vi "IVCurveCustom.vi"(7 "OriginalSweepInfo":T1, 8 "ReadExtra":bool=TRUE, 9 "SweepInfo":T1, 10 "Program":string, 11 "UiDefinition":T4) -> (1 "appended array":dbl[][](array[numeric]), 3 "InfoCluster":T2)   [LabVIEW 2020]
uses:
  UIReferences.ctl
  D:/LabviewDXFViewer/LabviewDXFViewer/bin/Release/LabviewDXFViewer.exe
  LabviewDXFViewer/bin/Release/LabviewDXFViewer.exe
  CapacitanceInfos.ctl
  CapacitanceRecord.ctl
  Keithley 2600 Series/Keithley 2600 Series.lvlib
panel:
  out "error out 4":errorcluster
  out "error out 3":errorcluster
  out "error out 2":errorcluster
  out "error out":errorcluster
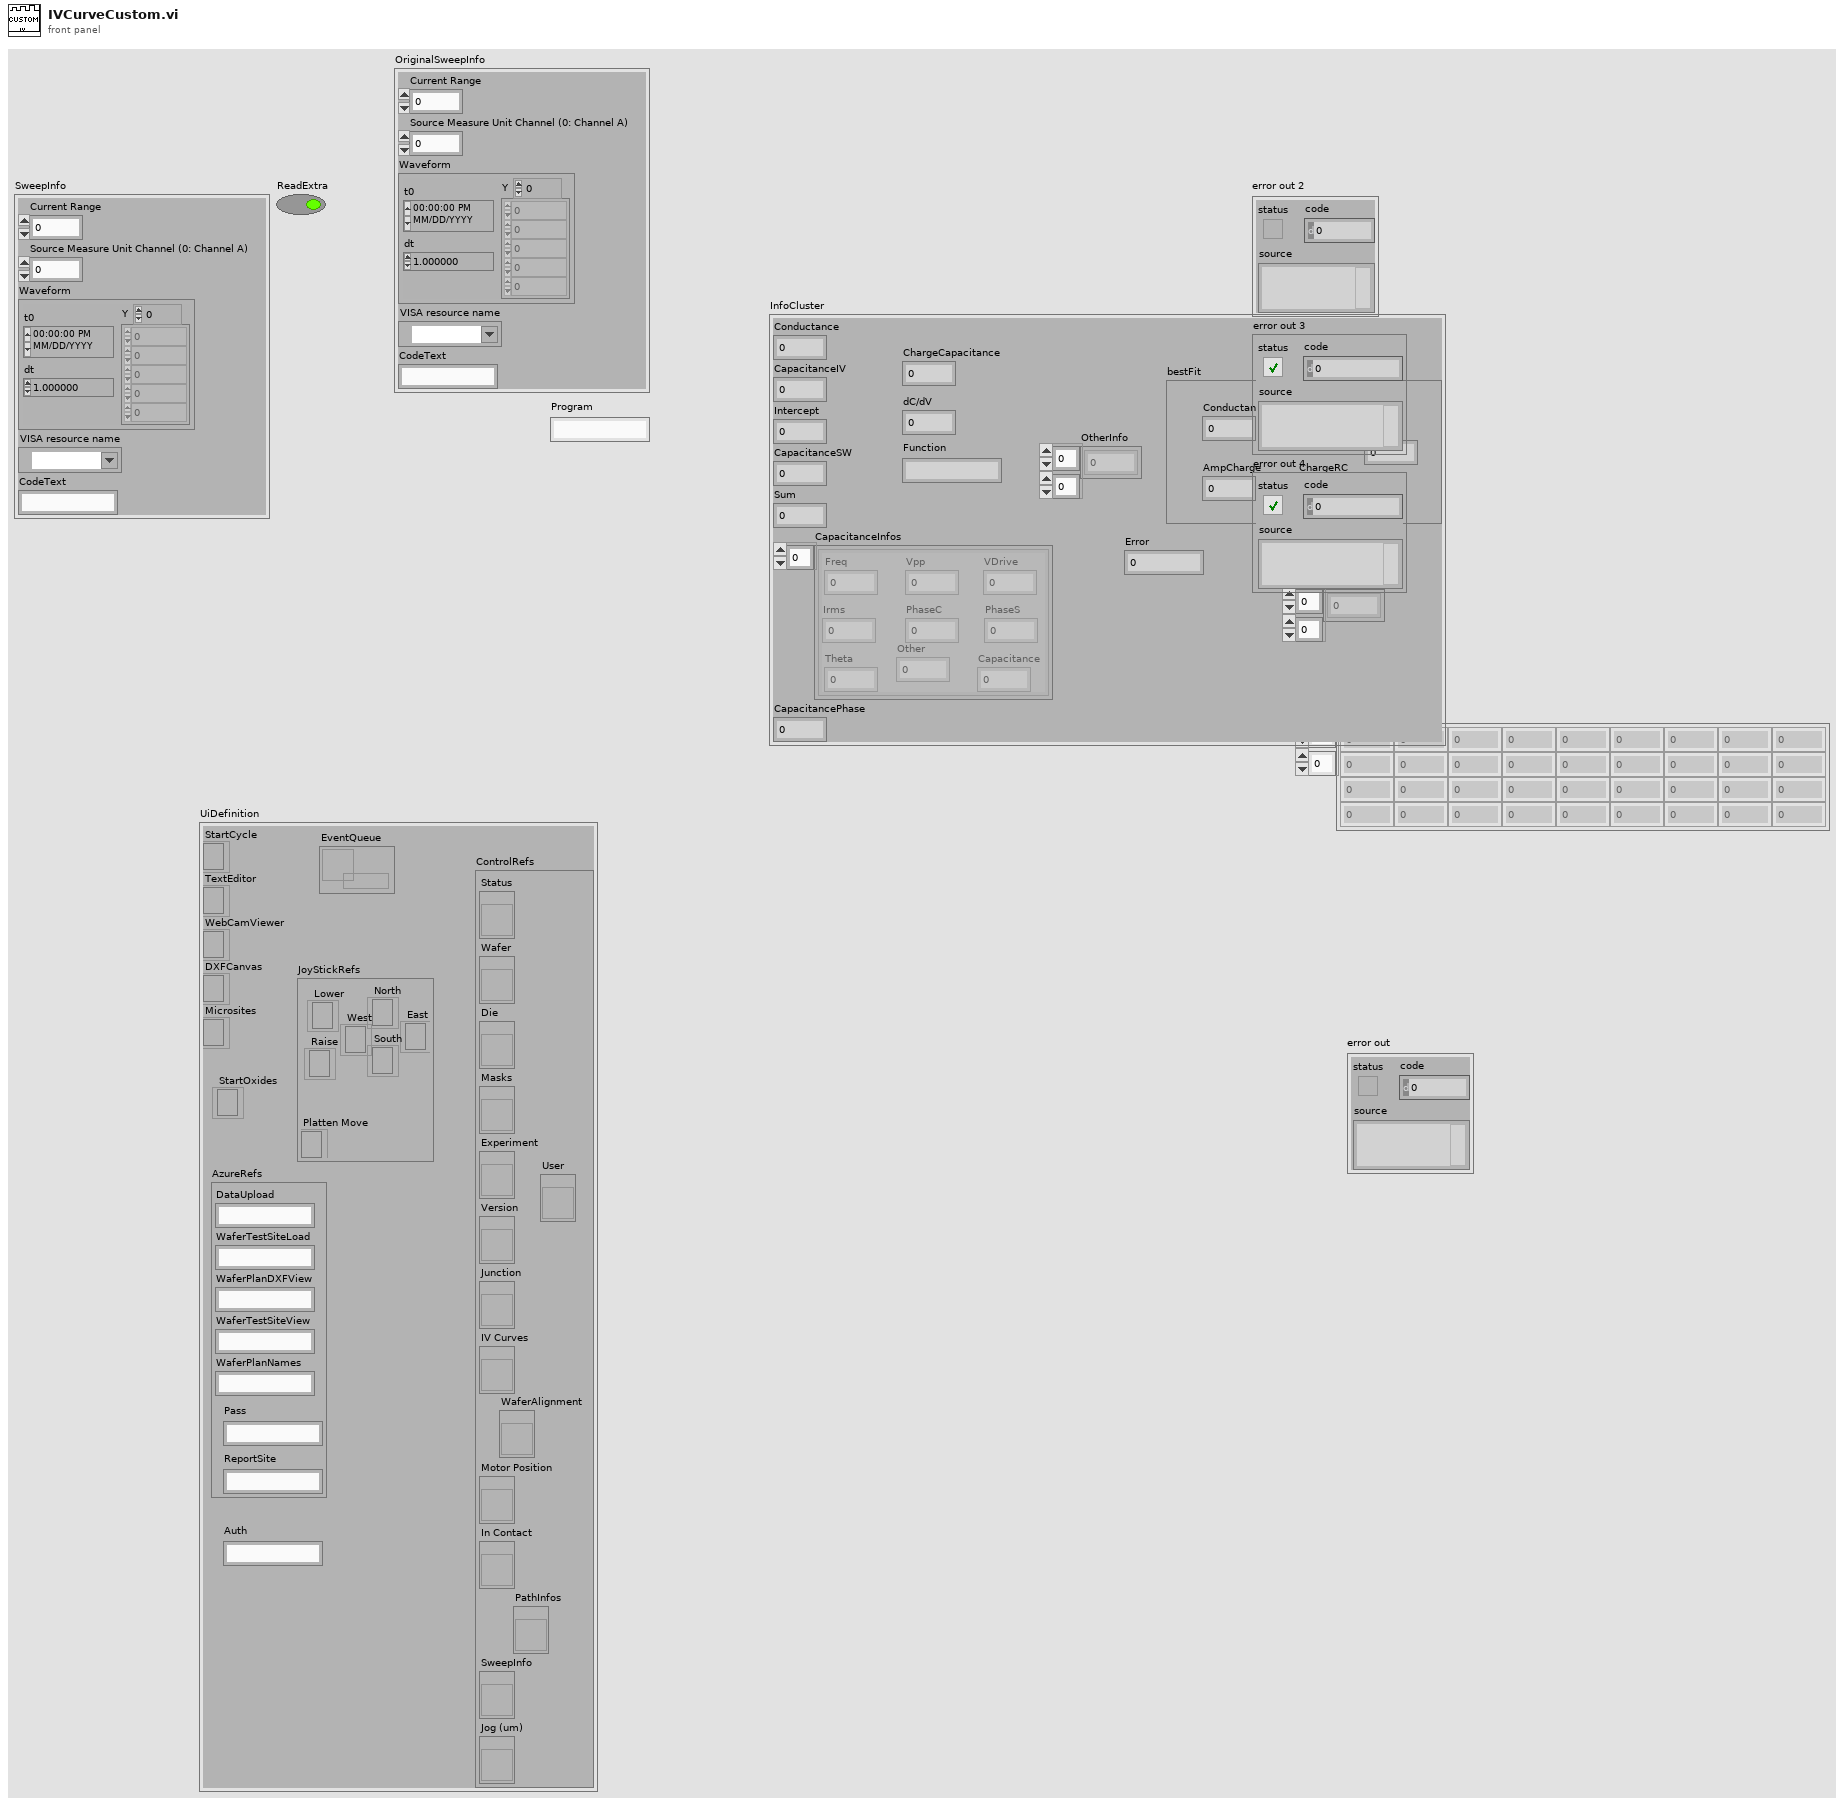
[diagram p1: front panel]
types:
  T1 = cluster{"Current Range":dbl, "Source Measure Unit Channel (0: Channel A)":i32, "Waveform":waveform(dbl), "VISA resource name":refnum<visa-resource-name>, "CodeText":string}
  T2 = typedef "CapacitanceInfos.ctl" = cluster{"Conductance":dbl, "CapacitanceIV":dbl, "Intercept":dbl, "CapacitanceSW":dbl, "Sum":dbl, "CapacitanceInfos":T3[], "CapacitancePhase":dbl, "dC/dV":dbl, "Function":string, "OtherInfo":dbl[][], "ChargeCapacitance":dbl, "FitCurves":dbl[][], "Error":dbl, "bestFit":cluster{"Conductance":dbl, "Current0":dbl, "AmpCharge":dbl, "ChargeRC":dbl, "V0":dbl}}
  T3 = typedef "CapacitanceRecord.ctl" = cluster{"Freq":dbl, "Vpp":dbl, "PhaseS":dbl, "Irms":dbl, "PhaseC":dbl, "Theta":dbl, "VDrive":dbl, "Capacitance":dbl, "Other":dbl}
  T4 = typedef "UIReferences.ctl" = cluster{"StartCycle":refnum<k24>, "TextEditor":refnum<k24>, "WebCamViewer":refnum<k24>, "DXFCanvas":refnum<k24>, "Microsites":refnum<k24>, "JoyStickRefs":cluster{"North":refnum<k24>, "Lower":refnum<k24>, "Raise":refnum<k24>, "Platten Move":refnum<k24>, "West":refnum<k24>, "East":refnum<k24>, "South":refnum<k24>}, "AzureRefs":cluster{"DataUpload":string, "WaferTestSiteLoad":string, "WaferPlanDXFView":string, "WaferTestSiteView":string, "WaferPlanNames":string, "Pass":string, "ReportSite":string}, "ControlRefs":cluster{"Status":refnum<vi>, "Wafer":refnum<vi>, "Die":refnum<vi>, "Masks":refnum<vi>, "Experiment":refnum<vi>, "Version":refnum<vi>, "Junction":refnum<vi>, "IV Curves":refnum<vi>, "Motor Position":refnum<vi>, "In Contact":refnum<vi>, "SweepInfo":refnum<vi>, "Jog (um)":refnum<vi>, "PathInfos":refnum<vi>, "User":refnum<vi>, "WaferAlignment":refnum<vi>}, "EventQueue":refnum<queue>, "StartOxides":refnum<k24>, "Auth":string}
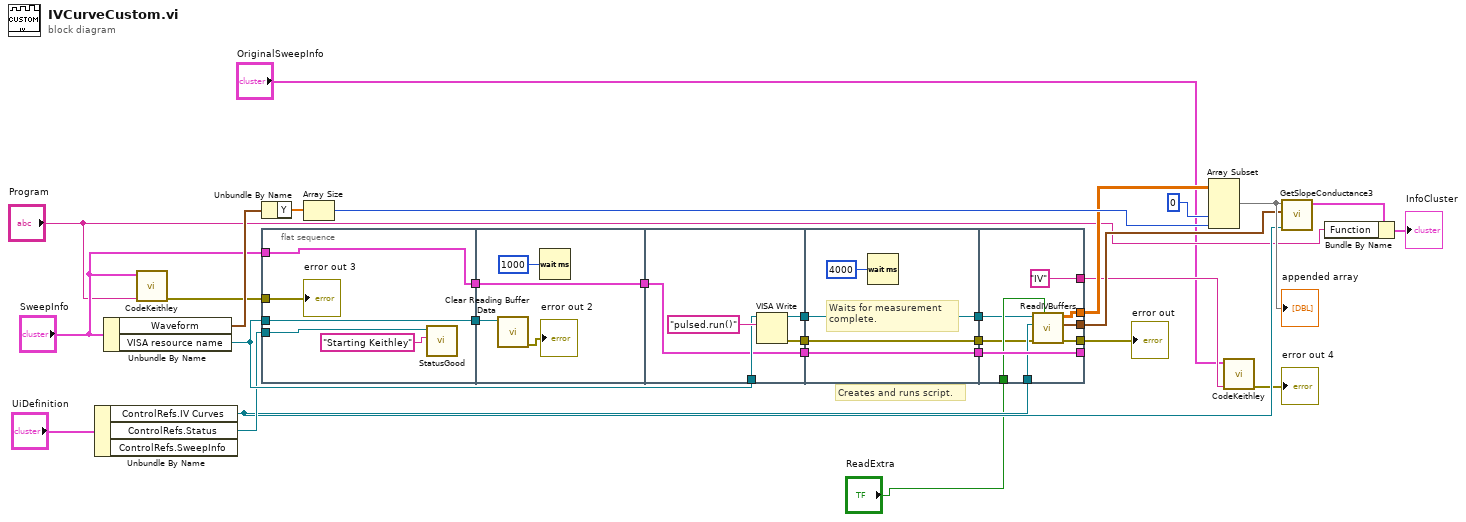
[diagram p0: block diagram]
diagram:
  # "Creates and runs script."
  n1 = Unbundle By Name("UiDefinition") -> ("ControlRefs.IV Curves"=w9:refnum<vi>, "ControlRefs.Status"=w21:refnum<vi>)  [unwired: 1 out]
  n2 = Unbundle By Name("SweepInfo") -> ("Waveform"=w27:waveform(dbl), "VISA resource name"=w28:refnum<visa-resource-name>)
  n3 = call "CodeKeithley.vi"("Program"="Program", "SweepInfo"="SweepInfo") -> ("error out"=w7:errorcluster)  [unwired: 9 in]
  n4 = Unbundle By Name(w27) -> ("Y"=w26:dbl[])
  n5 = flat-sequence {
    tunnel: w28 -> [w35]
    tunnel: [w35] -> w22
    tunnel: w21 -> [w34]
    tunnel: [w32] -> w20
    tunnel: "SweepInfo" -> [w32]
    tunnel: w7 -> [w31]
    tunnel: w22 -> [w38]
    tunnel: w20 -> [w36]
    tunnel: [w36] -> w17
    tunnel: [w42] -> w30
    tunnel: w28 -> [w43]
    tunnel: [w41] -> w18
    tunnel: w17 -> [w41]
    tunnel: [w40] -> w10
    tunnel: w30 -> [w48]
    tunnel: w18 -> [w46]
    tunnel: [w48] -> w16
    tunnel: [w46] -> w15
    tunnel: [w45] -> w11
    tunnel: w10 -> [w45]
    tunnel: [w57] -> _
    tunnel: w16 -> [w54]
    tunnel: w15 -> [w57]
    tunnel: "ReadExtra" -> [w56]
    tunnel: w9 -> [w55]
    tunnel: [w53] -> w14
    tunnel: [w52] -> w13
    tunnel: [w51] -> w12
    tunnel: w11 -> [w50]
    tunnel: ["IV" ("y")] -> w2
    frame #0 {
      n6 = call "StatusGood.vi"("Text.Text"="Starting Keithley", "String in"=w34) -> ()  [unwired: 10 in]
      "error out 3" <- w31
    }
    frame #1 {
      n7 = call "Clear Reading Buffer Data.vi"("VISA resource name"=w38) -> ("error out"=→"error out 2":errorcluster)  [unwired: 9 in, 1 out]
      n8 = Wait (ms)(milliseconds to wait=u32 1000) -> ()  [unwired: 1 out]
    }
    frame #2 {
      n9 = VISA Write(VISA resource name=w43, write buffer="pulsed.run()" ("format string")) -> (VISA resource name out=w42:refnum<visa-resource-name>, error out=w40:errorcluster)  [unwired: 1 in, 1 out]
    }
    frame #3 {
      # "Waits for measurement complete."
      n10 = Wait (ms)(milliseconds to wait=4000) -> ()  [unwired: 1 out]
    }
    frame #4 {
      n11 = call "ReadIVBuffers.vi"("GetCapacitors"=w56, "error in (no error)"=w50, "XYGraph Refnum"=w55, "VISA Refnum in"=w54) -> ("error out"=w53:errorcluster, "CapacitanceInfos"=w52:T3[], "Array"=w51:dbl[][])  [unwired: 5 in]
    }
  }
  n12 = Array Size(array=w26) -> (size(s)=w25:i32)
  n13 = Array Subset(array=w12, index (col)=0 ("index"), length (col)=w25) -> (w23:dbl[][])  [unwired: 2 in]
  "appended array" <- w23
  n14 = call "CodeKeithley.vi"("Program"=w2, "SweepInfo"="OriginalSweepInfo") -> ("error out"=→"error out 4":errorcluster)  [unwired: 9 in]
  n15 = call "GetSlopeConductance3.vi"("XYGraph Refnum"=w9, "CapacitanceRecords"=w13, "Array in"=w23) -> ("InfoCluster"=w6:T2)  [unwired: 7 in, 1 out]
  n16 = Bundle By Name(cluster=w6, "Function"="Program") -> (→"InfoCluster":T2)
  "error out" <- w14
